vi "Polynomial Plot (Samples).vi"(8 "P(x)":dbl[](array[numeric]), 11 "X":dbl[](array[numeric])) -> (0 "error":i32, 3 "polynomial plot":cluster{dbl[], "P(A)":dbl[]}(graph))   [LabVIEW 2020, in "NI_AALPro.lvlib"]
doc: "Plots the evaluations of polynomial <B>P(x)</B>. Wire data to the <B>X</B> input to determine the polymorphic instance to use or manually select the instance."
uses:
  NI_AALPro.lvlib
  1D Polynomial Evaluation (DBL).vi
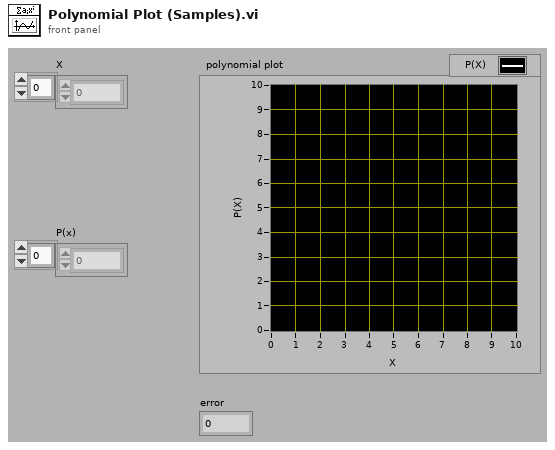
[diagram p1: front panel]
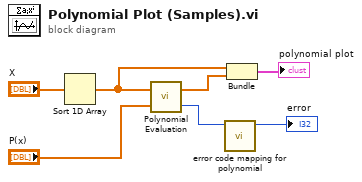
[diagram p0: block diagram]
diagram:
  n1 = Sort 1D Array(array="X") -> (sorted array=w4:dbl[])
  n2 = call-poly "Polynomial Evaluation.vi"("P(x)"="P(x)", "A"=w4) -> ("error"=w2:i32, "P(A)"=w6:dbl[])
  n3 = call "error code mapping for polynomial.vi"("error in"=w2) -> ("error out"=→"error":i32)  [unwired: 10 in]
  n4 = Bundle(w4, "P(A)"=w6) -> (→"polynomial plot":cluster{dbl[], "P(A)":dbl[]})  [unwired: 1 in]
